vi "Create Response.vi"(7 "error":bool, 8 "error in (no error)":errorcluster, 9 "JSON Tree In":variant, 10 "id value":string, 11 "jsonrpc":string) -> (0 "error out":errorcluster, 2 "id String":string, 3 "Response out":refnum<class "Response.lvclass">)   [LabVIEW 2015, in "Response.lvclass"]
uses:
  Response.lvclass
  id/id.lvclass
  New folder/result.lvclass
  error/error.lvclass
  Response.lvclass/Response.ctl
  JSONable/JSONable.lvclass
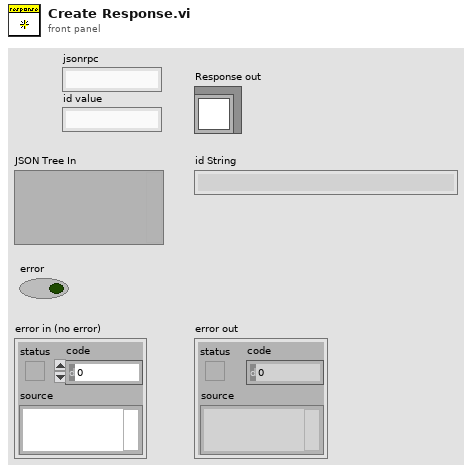
[diagram p1: front panel]
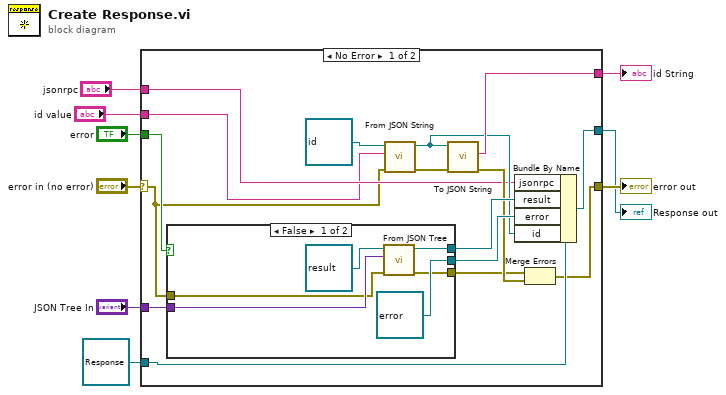
[diagram p0: block diagram]
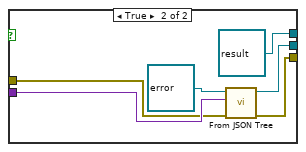
[diagram p2: hidden frame]
diagram:
  n1 = case shown="No Error" "error in (no error)" {
    selector: "error in (no error)" -> [w10 w39]
    tunnel: [w16 w39] -> w8
    tunnel: [w25 w38] -> w7
    tunnel: refnum<class "Response.lvclass"> refnum ("Response.lvclass") -> [w24 w38]
    tunnel: "JSON Tree In" -> [w23 _]
    tunnel: "error" -> [w21 _]
    tunnel: [w19 _] -> w3
    tunnel: "jsonrpc" -> [w12 _]
    tunnel: "id value" -> [w11 _]
    frame No Error {
      n2 = case shown="False" w21 {
        tunnel: w23 -> [w30 w37]
        tunnel: [w29 refnum<class "result.lvclass"> refnum ("result")] -> w22
        tunnel: [refnum<class "error.lvclass"> refnum ("error") w35] -> w20
        tunnel: [w26 w33] -> w17
        tunnel: w10 -> [w27 w32]
        frame False {
          n3 = call-dynamic "From JSON Tree.vi"("error in (no error)"=w27, "JSON Tree In"=w30, "result in"=refnum<class "result.lvclass"> refnum ("result")) -> ("error out"=w26:errorcluster, "result out"=w29:refnum<class "result.lvclass">)  [unwired: 7 in]
        }
        frame True {
          n4 = call-dynamic "From JSON Tree.vi"("error in (no error)"=w32, "JSON Tree In"=w37, "error in"=refnum<class "error.lvclass"> refnum ("error")) -> (0:"error out"=w33:errorcluster, 3:"error out"=w35:refnum<class "error.lvclass">)  [unwired: 7 in]
        }
      }
      n5 = call "From JSON String.vi"("error in (no error)"=w10, "JSON String"=w11, "JSONable in"=refnum<class "id.lvclass"> refnum ("id in")) -> ("error out"=w13:errorcluster, "JSONable out"=w14:refnum<class "id.lvclass">)  [unwired: 7 in]
      n6 = call "To JSON String.vi"("error in (no error)"=w13, "JSONable in"=w14) -> ("error out"=w18:errorcluster, "JSON String"=w19:string)  [unwired: 7 in, 1 out]
      n7 = Bundle By Name(cluster=w24, "jsonrpc"=w12, "result"=w22, "error"=w20, "id"=w14) -> (w25:refnum<class "Response.lvclass">)
      n8 = Merge Errors(w17, w18) -> (w16:errorcluster)
    }
    frame Error {
    }
  }
  "error out" <- w8
  "Response out" <- w7
  "id String" <- w3
